vi "Chnls2Pixel.vi"(10 "Secondary":i32, 11 "Primary":i32) -> (3 "Pixel ID":i8)   [LabVIEW 2016]
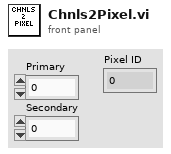
[diagram p1: front panel]
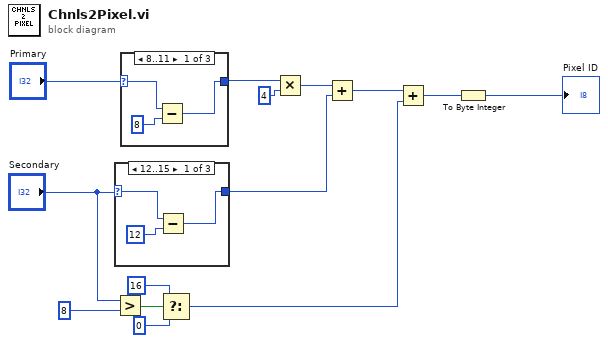
[diagram p0: block diagram]
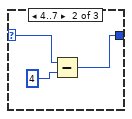
[diagram p2: hidden frame]
diagram:
  n1 = case shown="12..15" "Secondary" {
    selector: "Secondary" -> [w15 w18 _]
    tunnel: [w16 w19 _] -> w10
    frame 12..15 {
      n2 = Subtract(x=w15, y=12) -> (x-y=w16:i32)
    }
    frame 4..7 {
      n3 = Subtract(x=w18, y=4) -> (x-y=w19:i32)
    }
    frame Default {
    }
  }
  n4 = Greater?(x="Secondary", y=8) -> (0:w4:bool)
  n5 = case shown="8..11" "Primary" {
    selector: "Primary" -> [w21 w24 _]
    tunnel: [w22 w24 _] -> w13
    frame 8..11 {
      n6 = Subtract(x=w21, y=8) -> (x-y=w22:i32)
    }
    frame 0..3 {
    }
    frame Default {
    }
  }
  n7 = Select(t=16, s=w4, f=0) -> (s? t:f=w2:i32)
  n8 = Multiply(x=w13, y=4) -> (x*y=w11:i32)
  n9 = Add(x=w11, y=w10) -> (x+y=w6:i32)
  n10 = Add(x=w6, y=w2) -> (x+y=w5:i32)
  n11 = To Byte Integer(number=w5) -> (8bit integer=→"Pixel ID":i8)
